vi "CheckAndSaveFile.vi"(0 "new Table":string[][](array[string]), 1 "path":path) -> ()   [LabVIEW 2014]
uses:
  <vilib>/Utility/file.llb/Read From Spreadsheet File (string).vi
  <vilib>/Utility/file.llb/Write To Spreadsheet File (string).vi
panel:
  out "Array":bool[][](array[boolean])
  out "old Table":string[][](array[string])
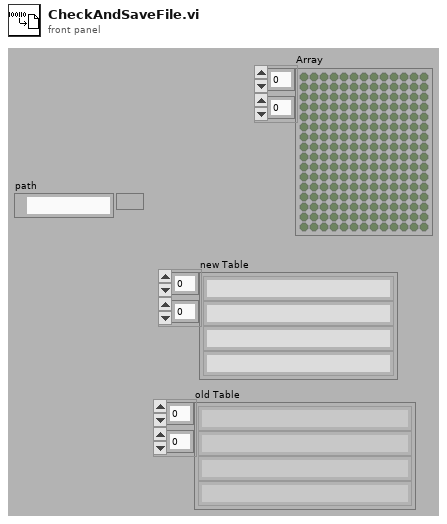
[diagram p1: front panel]
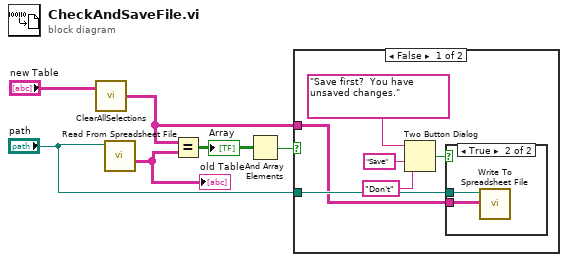
[diagram p0: block diagram]
diagram:
  n1 = call "ClearAllSelections.vi"("old Table"="new Table") -> ("New Table"=w4:string[][])
  n2 = call-poly <vilib>:"Read From Spreadsheet File.vi"("file path (dialog if empty)"="path") -> ("all rows"=w3:string[][])  [unwired: 6 in, 4 out]
  "old Table" <- w3
  n3 = Equal?(x=w4, y=w3) -> (x = y?=w2:bool[][])
  "Array" <- w2
  n4 = And Array Elements(Boolean array=w2) -> (logical AND=w1:bool)
  n5 = case shown="False" w1 {
    tunnel: "path" -> [w8 _]
    tunnel: w4 -> [w7 _]
    frame False {
      n6 = Two Button Dialog(message="Save first?  You have unsaved changes.", 1:"Don't" ("T button name (\"OK\")"), 2:"Save" ("T button name (\"OK\")")) -> (T button?=w9:bool)
      n7 = case shown="True" w9 {
        tunnel: w7 -> [_ w14]
        tunnel: w8 -> [_ w13]
        frame False {
        }
        frame True {
          n8 = call-poly <vilib>:"Write To Spreadsheet File.vi"("2D data"=w14, "file path (dialog if empty)"=w13) -> ()  [unwired: 6 in, 1 out]
        }
      }
    }
    frame True {
    }
  }
